vi "Send Immediate Stop Msg.vi"(8 "error in (no error)":errorcluster, 11 "Message Enqueuer":refnum<class "Message Enqueuer.lvclass">) -> (0 "error out":errorcluster)   [LabVIEW 2020, in "PriorityStopMessage.lvclass"]
doc: "此 VI 已过时，请使用 Send Priority Stop Msg.vi"
uses:
  PriorityStopMessage.lvclass
  <vilib>/ActorFramework/Message Enqueuer/Message Enqueuer.lvclass
  <vilib>/ActorFramework/Message Enqueuer/Message Priority.ctl
  <vilib>/ActorFramework/Stop Msg/Stop Msg.lvclass
  C:/Program Files/National Instruments/LabVIEW 2020/vi.lib/ActorFramework/Message/Message.lvclass
  <vilib>/ActorFramework/Message Enqueuer/Message Enqueuer.lvclass/Message Enqueuer.ctl
  <vilib>/ActorFramework/Message Priority Queue/Priority Enqueue.vi
panel:
  # "This method was not properly tested before pre-release!\nThe technique used here does not actually work and\nthere's no way around it with the current scoping of\nAF messaging resources. Your next best option is to use\nSend Priority Stop Msg with 'High' Priority."
  # "此方法在预发布之前没有经过适当的测试！\n这里使用的技术实际上不起作用\n根据目前的范围，这是无法避免的\nAF消息资源。你的下一个最佳选择是使用\n发送具有“高”优先级的优先级停止消息。"
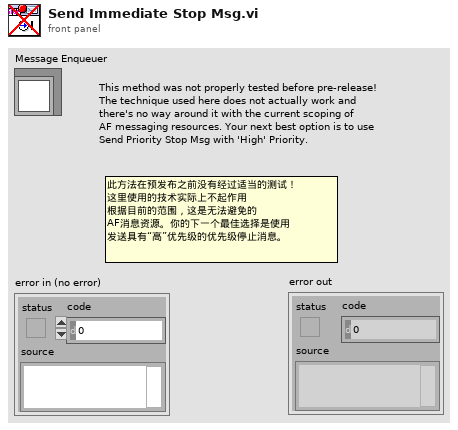
[diagram p1: front panel]
types:
  T1 = typedef "Actor Framework.lvlib/Message Enqueuer.lvclass/Message Priority.ctl" = enum16{"Low", "Normal", "High"}
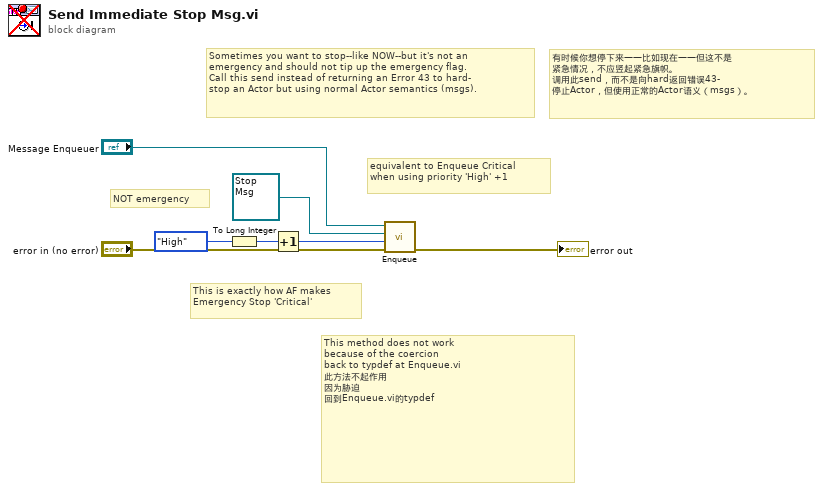
[diagram p0: block diagram]
diagram:
  # "有时候你想停下来——比如现在——但这不是\n紧急情况，不应竖起紧急旗帜。\n调用此send，而不是向hard返回错误43-\n停止Actor，但使用正常的Actor语义（msgs）。"
  # "This method does not work\nbecause of the coercion\nback to typdef at Enqueue.vi\n此方法不起作用\n因为胁迫\n回到Enqueue.vi的typdef"
  # "equivalent to Enqueue Critical\nwhen using priority 'High' +1"
  # "This is exactly how AF makes\nEmergency Stop 'Critical'"
  # "NOT emergency"
  # "Sometimes you want to stop--like NOW--but it's not an\nemergency and should not tip up the emergency flag.\nCall this send instead of returning an Error 43 to hard-\nstop an Actor but using normal Actor semantics (msgs)."
  n1 = To Long Integer(number=Message_Priority."High" ("Message Priority (Normal)")) -> (32bit integer=w1:i32)
  n2 = Increment(x=w1) -> (x+1=w2:i32)
  n3 = call <vilib>:"Enqueue.vi"("error in (no error)"="error in (no error)", "Message Priority (Normal)"=w2, "Message"=refnum<class "Stop Msg.lvclass"> refnum ("Actor Framework:Stop Msg"), "Message Enqueuer in"="Message Enqueuer") -> ("error out"=→"error out":errorcluster)  [unwired: 6 in, 1 out]
